vi "CollectDataQueue.vi"() -> (15 "CollectDataQueue":refnum<queue>)   [LabVIEW 2020, in "NI_DAQ.lvclass"]
uses:
  NI_DAQ.lvclass
  E:/01_Project/CXXXX/GKN/C18726_27program_191115004/software/DAQ/DAQ_operation_type.ctl
panel:
  out "波形图":dbl[][](graph)
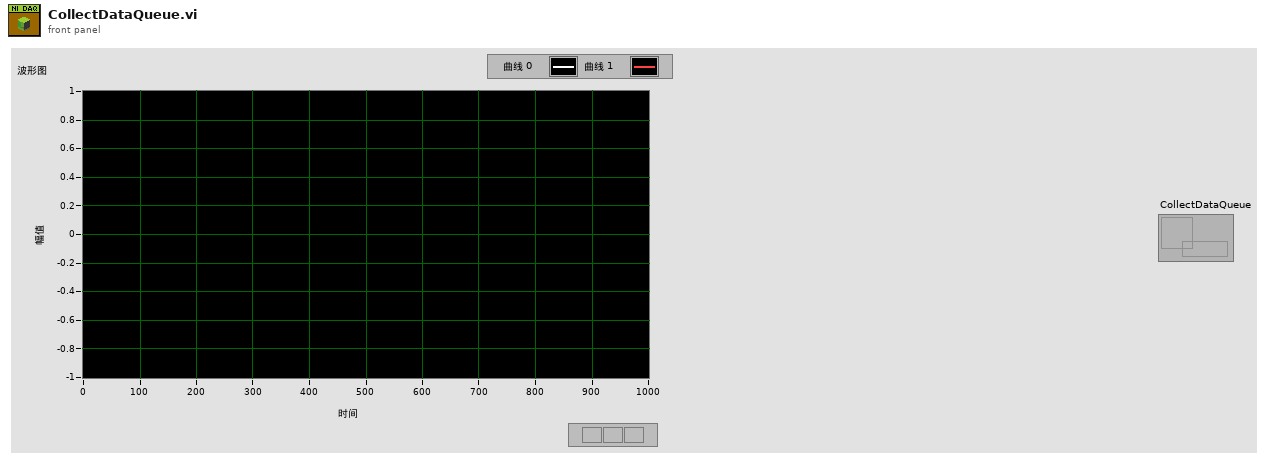
[diagram p1: front panel]
types:
  T1 = cluster{"real_data":dbl[][], "phys_data":dbl[][], "error_data":dbl[][]}
  T2 = typedef "DAQ_operation_type.ctl" = enum16{"idle", "read", "write", "clear", "init", "destroy"}
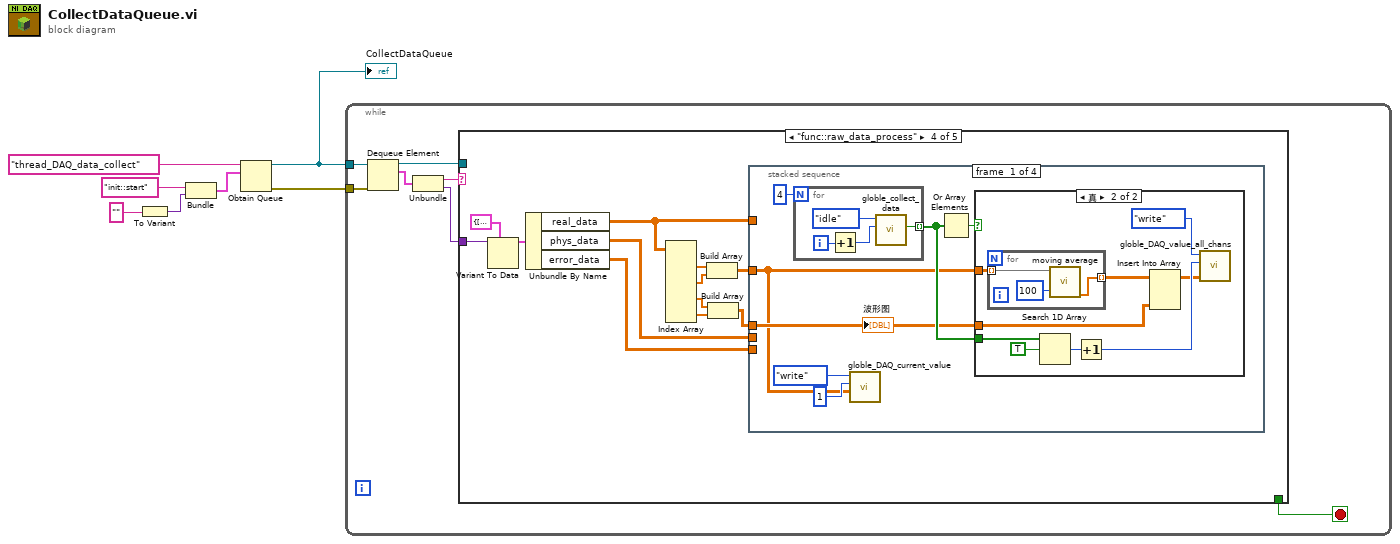
[diagram p0: block diagram]
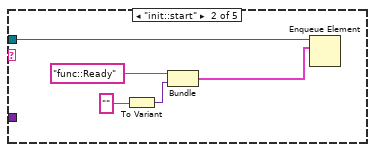
[diagram p3: hidden frame]
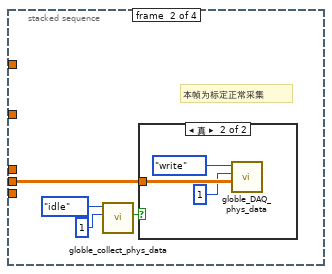
[diagram p6: hidden frame]
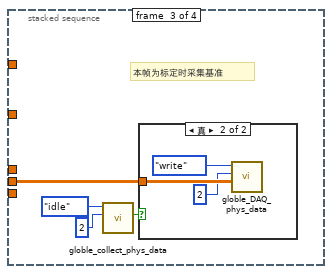
[diagram p8: hidden frame]
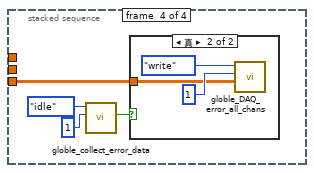
[diagram p10: hidden frame]
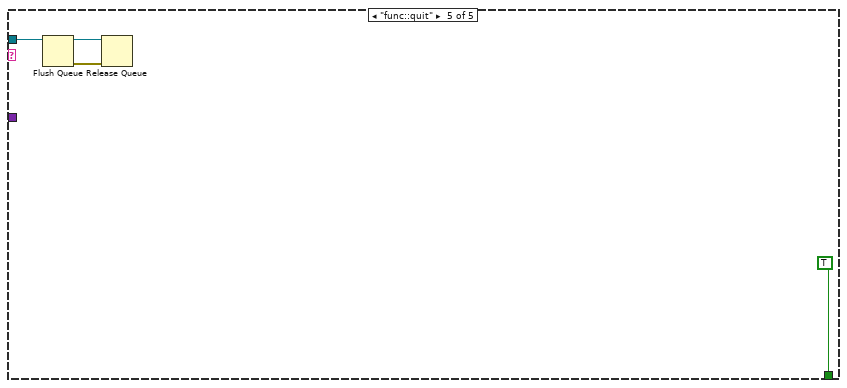
[diagram p12: hidden frame]
diagram:
  n1 = To Variant(anything="") -> (Variant=w6:variant)
  n2 = Bundle("init::start", "Variant"=w6) -> (w4:cluster{string, "Variant":variant})  [unwired: 1 in]
  n3 = Obtain Queue(name (unnamed)="thread_DAQ_data_collect" ("名称（未命名）"), element data type=w4) -> (queue out=w3:refnum<queue>, error out=w2:errorcluster)  [unwired: 3 in, 1 out]
  "CollectDataQueue" <- w3
  n4 = while {
    tunnel: w3 -> [w13]
    tunnel: w2 -> [w12]
    stop <- w8 stop-if-true
    n5 = Dequeue Element(queue=w13, error in (no error)=w12) -> (queue out=w9:refnum<queue>, element=w14:cluster{string, "Variant":variant})  [unwired: 1 in, 2 out]
    n6 = Unbundle(w14) -> (w11:string, "Variant"=w10:variant)
    n7 = case shown="\"func::raw_data_process\"" w11 {
      tunnel: w10 -> [_ _ _ w31 _]
      tunnel: w9 -> [_ w19 _ _ w77]
      tunnel: [_ _ _ _ TRUE] -> w8
      frame "Idle", Default {
      }
      frame "init::start" {
        n8 = To Variant(anything="") -> (Variant=w16:variant)
        n9 = Bundle("func::Ready", "Variant"=w16) -> (w15:cluster{string, "Variant":variant})  [unwired: 1 in]
        n10 = Enqueue Element(queue=w19, element=w15) -> ()  [unwired: 2 in, 3 out]
      }
      frame "func::Ready" {
      }
      frame "func::raw_data_process" {
        n11 = Variant To Data(type=T1 {"real_data"=[], "phys_data"=[], "error_data"=[]} ("输出簇"), Variant=w31) -> (data=w26:T1)  [unwired: 1 in, 1 out]
        n12 = Unbundle By Name(w26) -> ("real_data"=w25:dbl[][], "phys_data"=w21:dbl[][], "error_data"=w20:dbl[][])
        n13 = Index Array(array=w25) -> (element #1=w30:dbl[], element #2=w29:dbl[], element #3=w24:dbl[], element #4=w23:dbl[])  [unwired: 8 in]
        n14 = Build Array(w30, w29) -> (w28:dbl[][])
        n15 = Build Array(w24, w23) -> (w22:dbl[][])
        n16 = stacked-sequence {
          tunnel: w28 -> [w32 _ _ _]
          tunnel: w25 -> [_ _ _ _]
          tunnel: w21 -> [_ w56 w63 _]
          tunnel: w22 -> [w33 _ _ _]
          tunnel: w20 -> [_ _ _ w72]
          frame #0 {
            n17 = for {
              N: 4 -> [_]
              tunnel: [w40] -> w34 mode=indexing
              i -> [w41]
              n18 = Increment(x=w41) -> (x+1=w39:i32)
              n19 = call "globle_collect_data.vi"("chanel_nbr"=w39, "opearte"=DAQ_operation_type."idle") -> ("Collect_DAQ_data_out"=w40:bool)  [unwired: 8 in, 1 out]
            }
            n20 = call "globle_DAQ_current_value.vi"("data in"=w32, "chanel_nbr"=1, "opearte"=DAQ_operation_type."write") -> ()  [unwired: 7 in, 2 out]
            n21 = Or Array Elements(Boolean array=w34) -> (logical OR=w35:bool)
            n22 = case shown="真" w35 {
              tunnel: w32 -> [_ w50]
              tunnel: w34 -> [_ w47]
              tunnel: w33 -> [_ w44]
              frame False {
              }
              frame True {
                n23 = for {
                  tunnel: w50 -> [w54] mode=indexing
                  tunnel: [w52] -> w45 mode=indexing
                  n24 = call "moving average.vi"("Num"=100, "Filtered X"=w54) -> ("数组 2"=w52:dbl[])  [unwired: 9 in]
                }
                n25 = Search 1D Array(1D array=w47, element=TRUE) -> (index of element=w48:i32)  [unwired: 1 in]
                n26 = Increment(x=w48) -> (x+1=w46:i32)
                n27 = Insert Into Array(array=w45, new element=w44) -> (w43:dbl[][])  [unwired: 2 in]
                n28 = call "globle_DAQ_value_all_chans.vi"("data_in"=w43, "chanel_nbr"=w46, "opearte"=DAQ_operation_type."write") -> ()  [unwired: 6 in, 3 out]
              }
            }
            "波形图" <- w33
          }
          frame #1 {
            # "本帧为标定正常采集"
            n29 = call "globle_collect_phys_data.vi"("chanel_nbr"=1, "opearte"=DAQ_operation_type."idle") -> ("Collect_DAQ_data_out"=w55:bool)  [unwired: 8 in, 1 out]
            n30 = case shown="真" w55 {
              tunnel: w56 -> [_ w61]
              frame False {
              }
              frame True {
                n31 = call "globle_DAQ_phys_data.vi"("data_in"=w61, "chanel_nbr"=1, "opearte"=DAQ_operation_type."write") -> ()  [unwired: 7 in, 2 out]
              }
            }
          }
          frame #2 {
            # "本帧为标定时采集基准"
            n32 = call "globle_collect_phys_data.vi"("chanel_nbr"=2, "opearte"=DAQ_operation_type."idle") -> ("Collect_DAQ_data_out"=w62:bool)  [unwired: 8 in, 1 out]
            n33 = case shown="真" w62 {
              tunnel: w63 -> [_ w68]
              frame False {
              }
              frame True {
                n34 = call "globle_DAQ_phys_data.vi"("data_in"=w68, "chanel_nbr"=2, "opearte"=DAQ_operation_type."write") -> ()  [unwired: 7 in, 2 out]
              }
            }
          }
          frame #3 {
            n35 = call "globle_collect_error_data.vi"("chanel_nbr"=1, "opearte"=DAQ_operation_type."idle") -> ("Collect_DAQ_data_out"=w71:bool)  [unwired: 8 in, 1 out]
            n36 = case shown="真" w71 {
              tunnel: w72 -> [_ w73]
              frame False {
              }
              frame True {
                n37 = call "globle_DAQ_error_all_chans.vi"("data_in"=w73, "chanel_nbr"=1, "opearte"=DAQ_operation_type."write") -> ()  [unwired: 6 in, 3 out]
              }
            }
          }
        }
      }
      frame "func::quit" {
        n38 = Flush Queue(queue=w77) -> (queue out=w78:refnum<queue>, error out=w79:errorcluster)  [unwired: 1 in, 1 out]
        n39 = Release Queue(queue=w78, error in (no error)=w79) -> ()  [unwired: 1 in, 3 out]
      }
    }
  }
